vi "CAN_Receive.vi"(8 "错误输入（无错误）":errorcluster, 9 "WaitTime":i32, 10 "Length":u32, 11 "General_Input":T1={"DevType"=1, "DevIndex"=0, "CANIndex"=0} {"CANIndex" items=["0", "1"]; "DevType" items=["PCI5121"=1, "PCI9810"=2, "USBCAN1"=3, "USBCAN2"=4, "PCI9820"=5, "CAN232"=6, "PCI5110"=7, "CANLite(mini)"=8, "ISA9620"=9, "ISA5420"=10, "PC104CAN"=11, "CANETE"=12, "DNP9810"=13, "PCI9840B"=14, "PC104C2"=15, "PCI9820I"=16]}) -> (0 "错误输出":errorcluster, 2 "VCI_CAN_OBJ_R":T2 {"Reserved 2" format="%x"; "Reserved 1" format="%x"; "Reserved 0" format="%x"; "Data 7" format="%x"; "Data 6" format="%x"; "Data 5" format="%x"; "Data 4" format="%x"; "Data 3" format="%x"; "Data 2" format="%x"; "Data 1" format="%x"; "Data 0" format="%x"; "DataLen" format="%x"; "ExternFlag" format="%x"; "RemoteFlag" format="%x"; "SendType" format="%x"; "TimeFlag" format="%x"; "TimeStamp" format="%x"; "ID" format="%x"}, 3 "General_Output":T1={"DevType"=1, "DevIndex"=0, "CANIndex"=0} {"CANIndex" items=["0", "1"]; "DevType" items=["PCI5121"=1, "PCI9810"=2, "USBCAN1"=3, "USBCAN2"=4, "PCI9820"=5, "CAN232"=6, "PCI5110"=7, "CANLite(mini)"=8, "ISA9620"=9, "ISA5420"=10, "PC104CAN"=11, "CANETE"=12, "DNP9810"=13, "PCI9840B"=14, "PC104C2"=15, "PCI9820I"=16]})   [LabVIEW 2012]
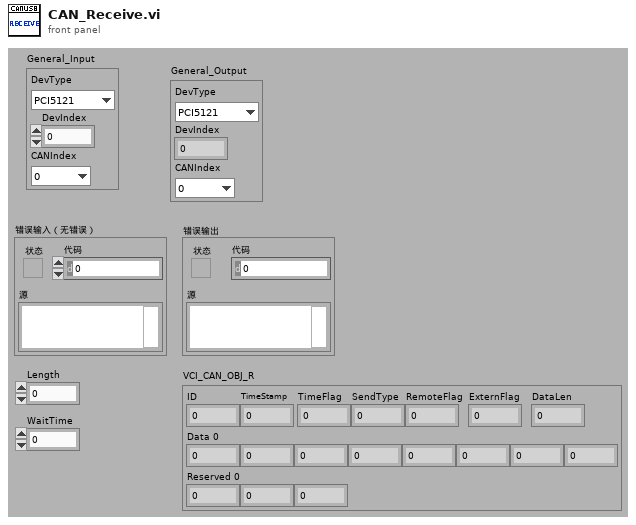
[diagram p1: front panel]
types:
  T1 = cluster{"DevType":u16, "DevIndex":u32, "CANIndex":u16}
  T2 = cluster{"ID":u32, "TimeStamp":u32, "TimeFlag":u8, "SendType":u8, "RemoteFlag":u8, "ExternFlag":u8, "DataLen":u8, "Data 0":u8, "Data 1":u8, "Data 2":u8, "Data 3":u8, "Data 4":u8, "Data 5":u8, "Data 6":u8, "Data 7":u8, "Reserved 0":u8, "Reserved 1":u8, "Reserved 2":u8}
  T3 = cluster{"DevType":u32, "DevIndex":u32, "CANIndex":u32}
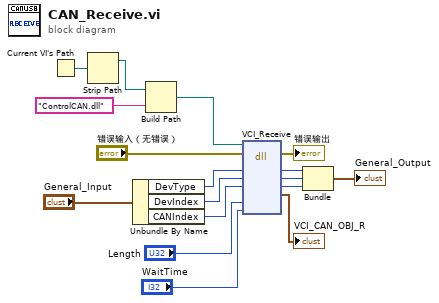
[diagram p0: block diagram]
diagram:
  n1 = Current VI's Path() -> (path=w10:path)
  n2 = Strip Path(path=w10) -> (stripped path=w11:path)  [unwired: 1 out]
  n3 = Unbundle By Name("General_Input") -> ("DevType"=w2:u16, "DevIndex"=w3:u32, "CANIndex"=w4:u16)
  n4 = Build Path(base path=w11, name or relative path="ControlCAN.dll" ("名称或相对路径")) -> (appended path=w1:path)
  n5 = dll-call lib="?" fn="VCI_Receive"(path in=w1, error in="错误输入（无错误）", "DevType"=w2, "DevIndex"=w3, "CANIndex"=w4, "Length"="Length", "WaitTime"="WaitTime") -> (error out=→"错误输出":errorcluster, "DevType"=w7:u32, "DevIndex"=w6:u32, "CANIndex"=w5:u32, "VCI_CAN_OBJ_R"=→"VCI_CAN_OBJ_R":T2)  [unwired: 5 in, 1 out]
  n6 = Bundle("DevType"=w7, "DevIndex"=w6, "CANIndex"=w5) -> (→"General_Output":T3)  [unwired: 1 in]
